vi "rectifi_string.vi"(10 "input":string) -> (2 "output":string)   [LabVIEW 2020]
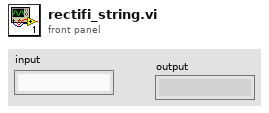
[diagram p1: front panel]
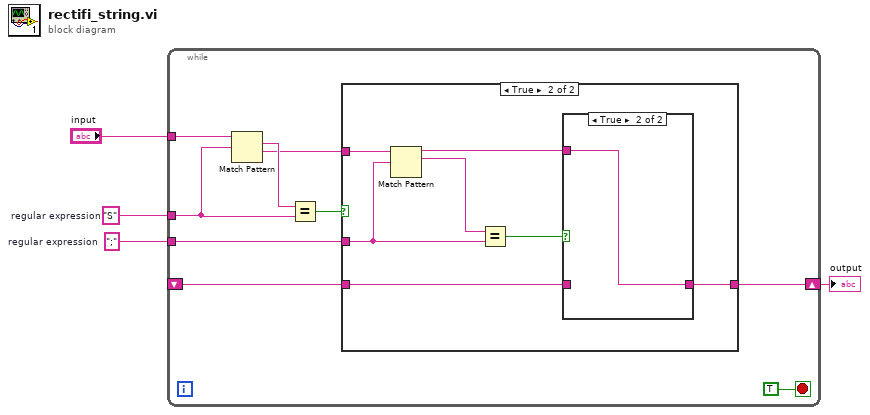
[diagram p0: block diagram]
diagram:
  w2 = ";"  # regular expression
  w3 = "S"  # regular expression
  n1 = while {
    tunnel: "input" -> [w13]
    tunnel: w3 -> [w11]
    tunnel: w2 -> [w8]
    shift-right: [w6] -> w1
    shift-left: _ -> [w5]
    stop <- TRUE stop-if-true
    n2 = Match Pattern(string=w13, regular expression=w11) -> (match substring=w12:string, after substring=w9:string)  [unwired: 1 in, 2 out]
    n3 = Equal?(x=w12, y=w11) -> (x = y?=w10:bool)
    n4 = case shown="True" w10 {
      tunnel: w9 -> [_ w21]
      tunnel: w8 -> [_ w20]
      tunnel: [w14 w16] -> w6
      tunnel: w5 -> [w14 w15]
      frame False {
      }
      frame True {
        n5 = Match Pattern(string=w21, regular expression=w20) -> (before substring=w17:string, match substring=w18:string)  [unwired: 1 in, 2 out]
        n6 = Equal?(x=w18, y=w20) -> (x = y?=w19:bool)
        n7 = case shown="True" w19 {
          tunnel: w17 -> [_ w23]
          tunnel: [w22 w23] -> w16
          tunnel: w15 -> [w22 _]
          frame False {
          }
          frame True {
          }
        }
      }
    }
  }
  "output" <- w1
